vi "write cache to tdms.vi"(8 "error in":errorcluster, 9 "output type order":T2[](array[typedef]), 10 "cache in":T1, 11 "tdms file in":refnum<k34>) -> (0 "error out":errorcluster, 2 "cache out":T1, 3 "tdms file out":refnum<k34>)   [LabVIEW 2013, in "TDMS datalogger runtime.lvclass"]
uses:
  TDMS datalogger runtime.lvclass
  <vilib>/NI/Tag Bus/tag/Data Type.ctl
  data cache.ctl
  <vilib>/NI/Tag Bus/tag/tag descriptor.lvclass
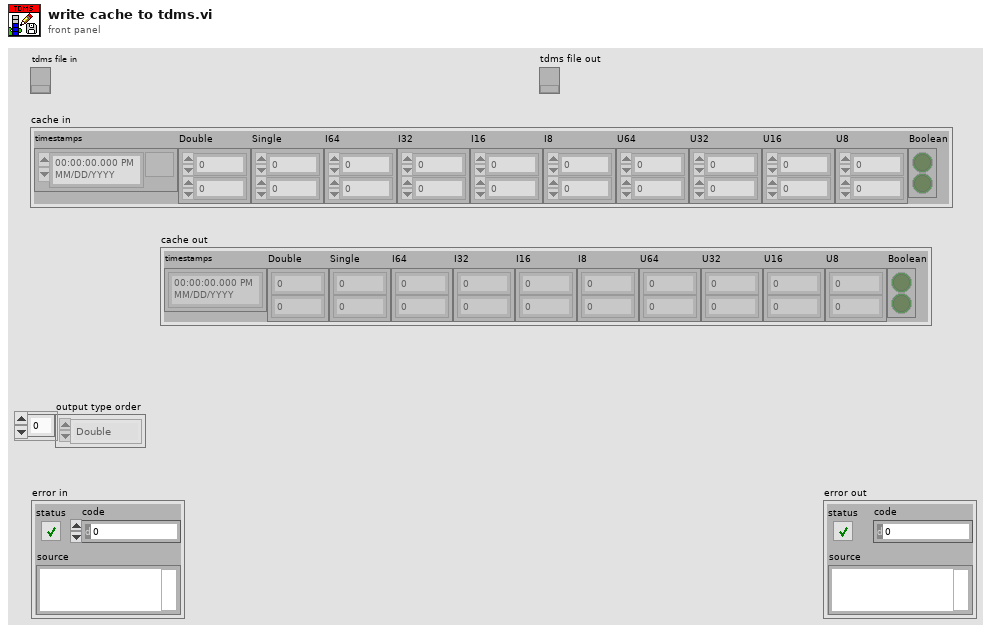
[diagram p1: front panel]
types:
  T1 = typedef "TDMS datalogger runtime.lvclass/data cache.ctl" = cluster{"timestamps":timestamp[], "Double":dbl[][], "Single":sgl[][], "I64":i64[][], "I32":i32[][], "I16":i16[][], "I8":i8[][], "U64":u64[][], "U32":u32[][], "U16":u16[][], "U8":u8[][], "Boolean":bool[][]}
  T2 = typedef "tag bus.lvlib/tag descriptor.lvclass/Data Type.ctl" = enum16{"Double", "Single", "I64", "I32", "I16", "I8", "U64", "U32", "U16", "U8", "Boolean", "String", "Array of Double", "Array of Single", "Array of I64", "Array of I32", "Array of I16", "Array of I8", "Array of U64", "Array of U32", "Array of U16", "Array of U8", "Array of Boolean", "Array of String"}
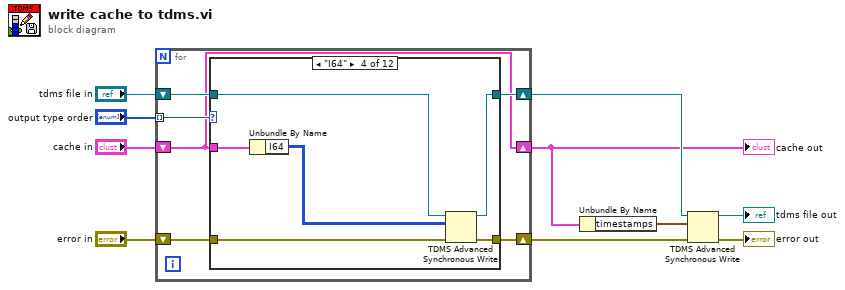
[diagram p0: block diagram]
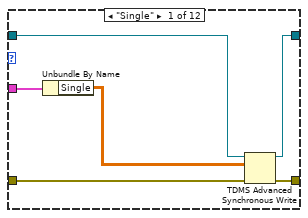
[diagram p2: hidden frame]
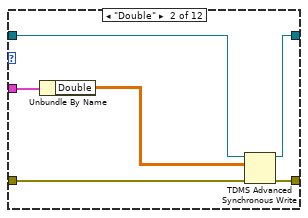
[diagram p3: hidden frame]
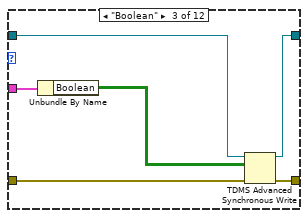
[diagram p4: hidden frame]
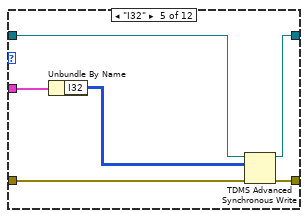
[diagram p5: hidden frame]
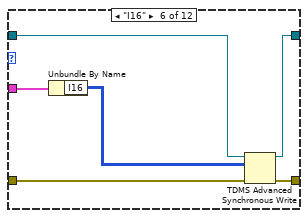
[diagram p6: hidden frame]
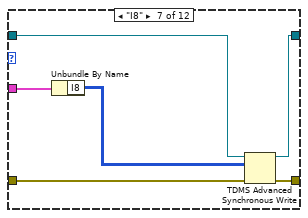
[diagram p7: hidden frame]
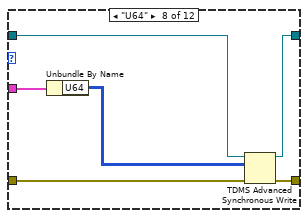
[diagram p8: hidden frame]
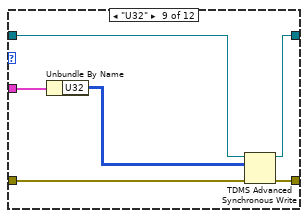
[diagram p9: hidden frame]
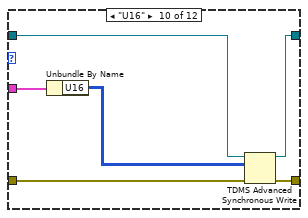
[diagram p10: hidden frame]
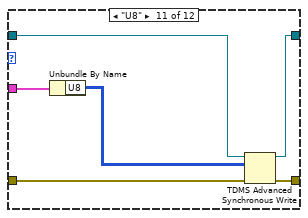
[diagram p11: hidden frame]
diagram:
  n1 = for {
    tunnel: "output type order" -> [w13] mode=indexing
    shift-right: [w14] -> w5
    shift-left: "error in" -> [w15]
    shift-right: [w12] -> w4
    shift-left: "tdms file in" -> [w16]
    shift-right: [w11] -> w3
    shift-left: "cache in" -> [w11]
    n2 = case shown="\"I64\"" w13 {
      tunnel: w16 -> [w22 w28 w34 w40 w46 w52 w58 w64 w70 w76 w82 w83]
      tunnel: w15 -> [w21 w27 w33 w39 w45 w51 w57 w63 w69 w75 w81 w84]
      tunnel: [w20 w26 w32 w38 w44 w50 w56 w62 w68 w74 w80 w84] -> w14
      tunnel: w11 -> [w19 w25 w31 w37 w43 w49 w55 w61 w67 w73 w79 _]
      tunnel: [w17 w23 w29 w35 w41 w47 w53 w59 w65 w71 w77 w83] -> w12
      frame "Single" {
        n3 = Unbundle By Name(w19) -> ("Single"=w18:sgl[][])
        n4 = TDMS Advanced Synchronous Write(8:w21, 10:w18, 11:w22) -> (0:w20:errorcluster, 3:w17:refnum<k34>)
      }
      frame "Double" {
        n5 = Unbundle By Name(w25) -> ("Double"=w24:dbl[][])
        n6 = TDMS Advanced Synchronous Write(8:w27, 10:w24, 11:w28) -> (0:w26:errorcluster, 3:w23:refnum<k34>)
      }
      frame "Boolean" {
        n7 = Unbundle By Name(w31) -> ("Boolean"=w30:bool[][])
        n8 = TDMS Advanced Synchronous Write(8:w33, 10:w30, 11:w34) -> (0:w32:errorcluster, 3:w29:refnum<k34>)
      }
      frame "I64" {
        n9 = Unbundle By Name(w37) -> ("I64"=w36:i64[][])
        n10 = TDMS Advanced Synchronous Write(8:w39, 10:w36, 11:w40) -> (0:w38:errorcluster, 3:w35:refnum<k34>)
      }
      frame "I32" {
        n11 = Unbundle By Name(w43) -> ("I32"=w42:i32[][])
        n12 = TDMS Advanced Synchronous Write(8:w45, 10:w42, 11:w46) -> (0:w44:errorcluster, 3:w41:refnum<k34>)
      }
      frame "I16" {
        n13 = Unbundle By Name(w49) -> ("I16"=w48:i16[][])
        n14 = TDMS Advanced Synchronous Write(8:w51, 10:w48, 11:w52) -> (0:w50:errorcluster, 3:w47:refnum<k34>)
      }
      frame "I8" {
        n15 = Unbundle By Name(w55) -> ("I8"=w54:i8[][])
        n16 = TDMS Advanced Synchronous Write(8:w57, 10:w54, 11:w58) -> (0:w56:errorcluster, 3:w53:refnum<k34>)
      }
      frame "U64" {
        n17 = Unbundle By Name(w61) -> ("U64"=w60:u64[][])
        n18 = TDMS Advanced Synchronous Write(8:w63, 10:w60, 11:w64) -> (0:w62:errorcluster, 3:w59:refnum<k34>)
      }
      frame "U32" {
        n19 = Unbundle By Name(w67) -> ("U32"=w66:u32[][])
        n20 = TDMS Advanced Synchronous Write(8:w69, 10:w66, 11:w70) -> (0:w68:errorcluster, 3:w65:refnum<k34>)
      }
      frame "U16" {
        n21 = Unbundle By Name(w73) -> ("U16"=w72:u16[][])
        n22 = TDMS Advanced Synchronous Write(8:w75, 10:w72, 11:w76) -> (0:w74:errorcluster, 3:w71:refnum<k34>)
      }
      frame "U8" {
        n23 = Unbundle By Name(w79) -> ("U8"=w78:u8[][])
        n24 = TDMS Advanced Synchronous Write(8:w81, 10:w78, 11:w82) -> (0:w80:errorcluster, 3:w77:refnum<k34>)
      }
      frame Default {
      }
    }
  }
  "cache out" <- w3
  n25 = Unbundle By Name(w3) -> ("timestamps"=w2:timestamp[])
  n26 = TDMS Advanced Synchronous Write(8:w5, 10:w2, 11:w4) -> (0:→"error out":errorcluster, 3:→"tdms file out":refnum<k34>)
